vi "createDeviceData.vi"(8 "error in (no error)":errorcluster, 11 "AoDeviceData in":refnum<class "AoDeviceData.lvclass">) -> (0 "error out":errorcluster, 3 "AoDeviceData out":refnum<class "AoDeviceData.lvclass">)   [LabVIEW 2011, in "DataMappers.lvlib" / "AoDeviceData.lvclass"]
uses:
  AoDeviceData.lvclass
  Hal/Channels/VoltOutput/AnalogOutput.lvclass
  AoDeviceData.lvclass/AoDeviceData.ctl
  DeviceData.lvclass
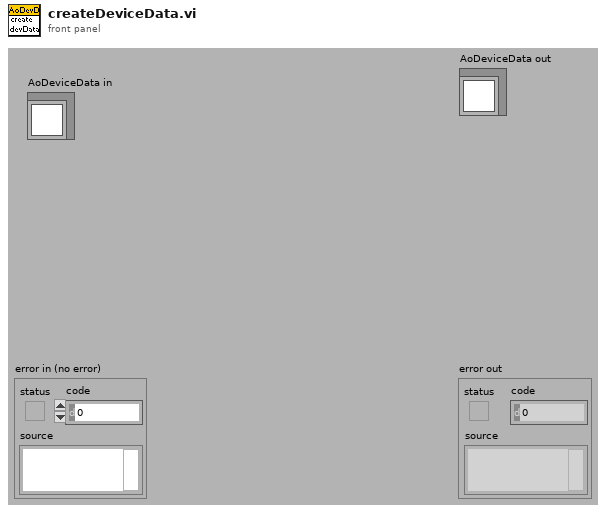
[diagram p1: front panel]
types:
  T1 = cluster{"Clock source":string, "Clock rate":dbl, "Start trigger line":string, "Sample Rate":dbl, "Sample No.":dbl}
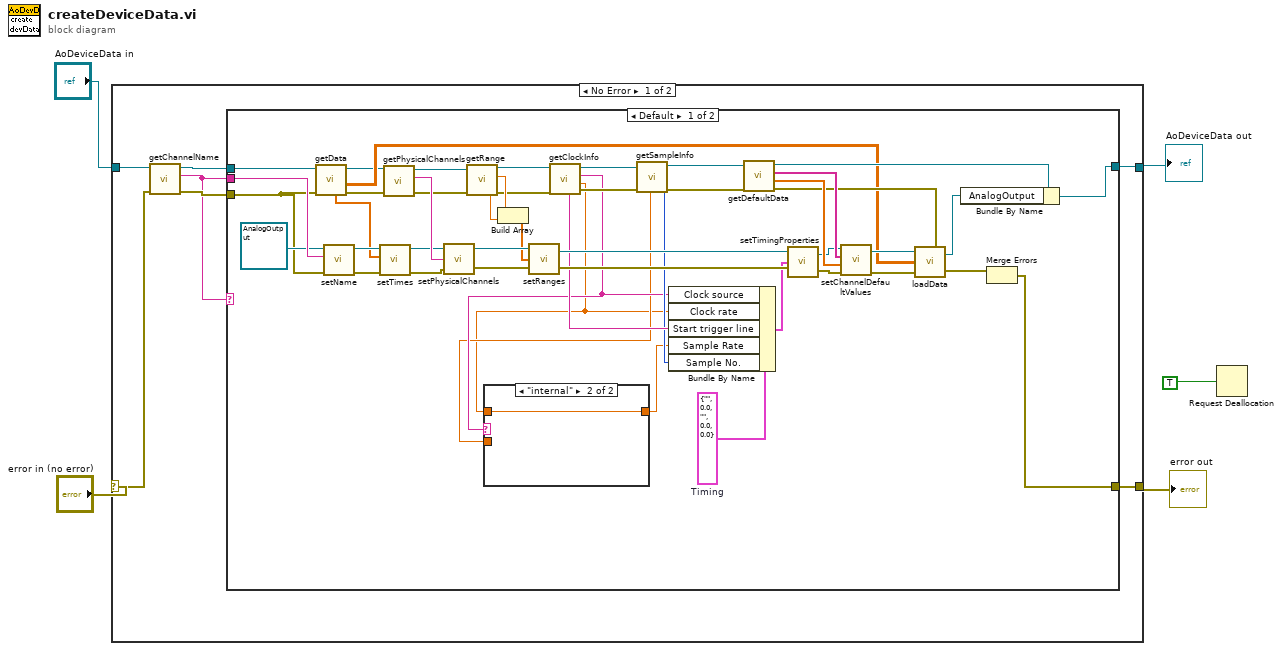
[diagram p0: block diagram]
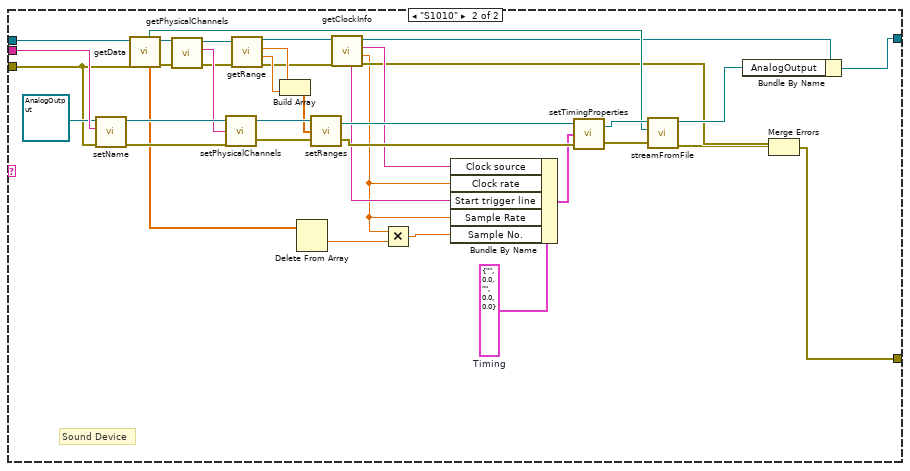
[diagram p3: hidden frame]
diagram:
  n1 = case shown="No Error" "error in (no error)" {
    selector: "error in (no error)" -> [w11 w100]
    tunnel: [w9 w101] -> w2
    tunnel: "AoDeviceData in" -> [w12 w101]
    tunnel: [w10 w100] -> w3
    frame No Error {
      n2 = call "getChannelName.vi"("error in (no error)"=w11, "DeviceData in"=w12) -> ("error out"=w7:errorcluster, "channelName"=w6:string, "DeviceData out"=w8:refnum<class "AoDeviceData.lvclass">)  [unwired: 7 in]
      n3 = case shown="Default" w6 {
        tunnel: w6 -> [w60 w99]
        tunnel: [w32 w79] -> w10
        tunnel: [w31 w69] -> w9
        tunnel: w8 -> [w26 w76]
        tunnel: w7 -> [w25 w77]
        frame Default {
          w44 = T1 {"Clock source"="", "Clock rate"=0.0, "Start trigger line"="", "Sample Rate"=0.0, "Sample No."=0.0}  # Timing
          n4 = call "getData.vi"("error in (no error)"=w25, "DeviceData in"=w26) -> ("error out"=w27:errorcluster, "dataArray"=w24:dbl[][], "DeviceData out"=w23:refnum<class "AoDeviceData.lvclass">, "times"=w13:dbl[])  [unwired: 4 in, 2 out]
          n5 = call "setName.vi"("error in (no error)"=w25, "name"=w60, "AnalogOutput.lvclass in"=refnum<class "AnalogOutput.lvclass"> refnum ("Hardware:Channels.lvlib:AnalogOutput.lvclass")) -> ("error out"=w16:errorcluster, "AnalogOutput.lvclass out"=w17:refnum<class "AnalogOutput.lvclass">)  [unwired: 7 in]
          n6 = call "setTimes.vi"("error in (no error)"=w16, "times"=w13, "AnalogOutput in"=w17) -> ("error out"=w15:errorcluster, "AnalogOutput out"=w14:refnum<class "AnalogOutput.lvclass">)  [unwired: 7 in]
          n7 = call "getPhysicalChannels.vi"("error in (no error)"=w27, "DeviceData in"=w23) -> ("error out"=w54:errorcluster, "physicalChannels"=w58:string, "DeviceData out"=w55:refnum<class "AoDeviceData.lvclass">)  [unwired: 7 in]
          n8 = call-dynamic "setPhysicalChannels.vi"("error in (no error)"=w15, "Physical Channels"=w58, "AnalogOutput.lvclass in"=w14) -> ("error out"=w56:errorcluster, "AnalogOutput.lvclass out"=w57:refnum<class "AnalogOutput.lvclass">)
          n9 = call "getRange.vi"("error in (no error)"=w54, "AoDeviceData in"=w55) -> ("error out"=w49:errorcluster, "max"=w53:dbl, "min"=w52:dbl, "AoDeviceData out"=w50:refnum<class "AoDeviceData.lvclass">)  [unwired: 6 in]
          n10 = Build Array(w52, w53) -> (w51:dbl[])
          n11 = call "setRanges.vi"("error in (no error)"=w56, "Ranges"=w51, "AnalogOutput.lvclass in"=w57) -> ("error out"=w47:errorcluster, "AnalogOutput.lvclass out"=w48:refnum<class "AnalogOutput.lvclass">)
          n12 = call "getClockInfo.vi"("error in (no error)"=w49, "DeviceData in"=w50) -> ("error out"=w45:errorcluster, "masterClockRate"=w19:dbl, "clock"=w21:string, "DeviceData out"=w46:refnum<class "AoDeviceData.lvclass">, "start_trigger"=w43:string)  [unwired: 5 in]
          n13 = call-dynamic "getSampleInfo.vi"("error in (no error)"=w45, "DeviceData in"=w46) -> ("error out"=w40:errorcluster, "sampleRate"=w20:dbl, "sampleNumber"=w22:i32, "DeviceData out"=w41:refnum<class "AoDeviceData.lvclass">)  [unwired: 6 in]
          n14 = case shown="\"internal\"" w21 {
            tunnel: w20 -> [w61 _]
            tunnel: w19 -> [_ w62]
            tunnel: [w61 w62] -> w18
            frame Default {
            }
            frame "internal" {
            }
          }
          n15 = Bundle By Name(cluster=w44, "Clock source"=w21, "Clock rate"=w19, "Start trigger line"=w43, "Sample Rate"=w18, "Sample No."=w22) -> (w42:T1)
          n16 = call "getDefaultData.vi"("error in (no error)"=w40, "DeviceData in"=w41) -> ("error out"=w28:errorcluster, "calibratedValues"=w37:dbl[], "channelAddresses"=w38:string[], "DeviceData out"=w29:refnum<class "AoDeviceData.lvclass">)  [unwired: 6 in]
          n17 = call "setTimingProperties.vi"("error in (no error)"=w47, "Timing"=w42, "AnalogOutput.lvclass in"=w48) -> ("error out"=w39:errorcluster, "AnalogOutput.lvclass out"=w36:refnum<class "AnalogOutput.lvclass">)
          n18 = call "setChannelDefaultValues.vi"("error in (no error)"=w39, "calibratedValues"=w37, "channel_addresses"=w38, "AnalogOutput in"=w36) -> ("error out"=w34:errorcluster, "AnalogOutput out"=w35:refnum<class "AnalogOutput.lvclass">)  [unwired: 6 in]
          n19 = call-dynamic "loadData.vi"("error in (no error)"=w34, "Data"=w24, "AnalogOutput in"=w35) -> ("error out"=w33:errorcluster, "AnalogOutput out"=w30:refnum<class "AnalogOutput.lvclass">)
          n20 = Bundle By Name(cluster=w29, "AnalogOutput"=w30) -> (w31:refnum<class "AoDeviceData.lvclass">)
          n21 = Merge Errors(w28, w33) -> (w32:errorcluster)
        }
        frame "S1010" {
          w83 = T1 {"Clock source"="", "Clock rate"=0.0, "Start trigger line"="", "Sample Rate"=0.0, "Sample No."=0.0}  # Timing
          # "Sound Device"
          n22 = call "setName.vi"("error in (no error)"=w77, "name"=w99, "AnalogOutput.lvclass in"=refnum<class "AnalogOutput.lvclass"> refnum ("Hardware:Channels.lvlib:AnalogOutput.lvclass")) -> ("error out"=w96:errorcluster, "AnalogOutput.lvclass out"=w97:refnum<class "AnalogOutput.lvclass">)  [unwired: 7 in]
          n23 = call "getData.vi"("error in (no error)"=w77, "DeviceData in"=w76) -> ("error out"=w78:errorcluster, "DeviceData out"=w75:refnum<class "AoDeviceData.lvclass">, "times"=w66:dbl[], "soundStreamPath"=w72:path)  [unwired: 4 in, 2 out]
          n24 = call "getPhysicalChannels.vi"("error in (no error)"=w78, "DeviceData in"=w75) -> ("error out"=w91:errorcluster, "physicalChannels"=w95:string, "DeviceData out"=w92:refnum<class "AoDeviceData.lvclass">)  [unwired: 7 in]
          n25 = call-dynamic "setPhysicalChannels.vi"("error in (no error)"=w96, "Physical Channels"=w95, "AnalogOutput.lvclass in"=w97) -> ("error out"=w93:errorcluster, "AnalogOutput.lvclass out"=w94:refnum<class "AnalogOutput.lvclass">)
          n26 = call "getRange.vi"("error in (no error)"=w91, "AoDeviceData in"=w92) -> ("error out"=w86:errorcluster, "max"=w90:dbl, "min"=w89:dbl, "AoDeviceData out"=w87:refnum<class "AoDeviceData.lvclass">)  [unwired: 6 in]
          n27 = Build Array(w89, w90) -> (w88:dbl[])
          n28 = Delete From Array(array=w66) -> (deleted portion=w64:dbl)  [unwired: 2 in, 1 out]
          n29 = call "setRanges.vi"("error in (no error)"=w93, "Ranges"=w88, "AnalogOutput.lvclass in"=w94) -> ("error out"=w84:errorcluster, "AnalogOutput.lvclass out"=w85:refnum<class "AnalogOutput.lvclass">)
          n30 = call "getClockInfo.vi"("error in (no error)"=w86, "DeviceData in"=w87) -> ("error out"=w68:errorcluster, "masterClockRate"=w65:dbl, "clock"=w82:string, "DeviceData out"=w70:refnum<class "AoDeviceData.lvclass">, "start_trigger"=w81:string)  [unwired: 5 in]
          n31 = Multiply(x=w65, y=w64) -> (x*y=w63:dbl)
          n32 = Bundle By Name(cluster=w83, "Clock source"=w82, "Clock rate"=w65, "Start trigger line"=w81, "Sample Rate"=w65, "Sample No."=w63) -> (w80:T1)
          n33 = call "setTimingProperties.vi"("error in (no error)"=w84, "Timing"=w80, "AnalogOutput.lvclass in"=w85) -> ("error out"=w73:errorcluster, "AnalogOutput.lvclass out"=w74:refnum<class "AnalogOutput.lvclass">)
          n34 = call-dynamic "streamFromFile.vi"("error in (no error)"=w73, "Path"=w72, "AnalogOutput in"=w74) -> ("error out"=w67:errorcluster, "AnalogOutput out"=w71:refnum<class "AnalogOutput.lvclass">)  [unwired: 7 in]
          n35 = Bundle By Name(cluster=w70, "AnalogOutput"=w71) -> (w69:refnum<class "AoDeviceData.lvclass">)
          n36 = Merge Errors(w68, w67) -> (w79:errorcluster)
        }
      }
    }
    frame Error {
    }
  }
  "error out" <- w3
  "AoDeviceData out" <- w2
  n37 = Request Deallocation(TRUE) -> ()
